vi "First Step.vi"(8 "error in (no error)":errorcluster, 11 "Magnetic Field Lakeshore Continuous.lvclass in":refnum<class "Magnetic Field Lakeshore Continuous.lvclass">) -> (0 "error out":errorcluster, 2 "Current Position":dbl, 3 "Magnetic Field Lakeshore Continuous.lvclass out":refnum<class "Magnetic Field Lakeshore Continuous.lvclass">)   [LabVIEW 2023, in "Magnetic Field Lakeshore Continuous.lvclass"]
doc: "(Dynamic) Reset the instrument and prepare to scan. Go to step #0 - the first step. If desired, the scanner may do this in a different way than usual (i.e. by preparing to move a long distance, or reset to home position.)"
uses:
  Magnetic Field Lakeshore Continuous.lvclass
  Magnetic Field Lakeshore Continuous.lvclass/Magnetic Field Lakeshore Continuous.ctl
  Scanner/Scanner.lvclass
  Instruments/Utility Classes/Scannable/Scannable.lvclass
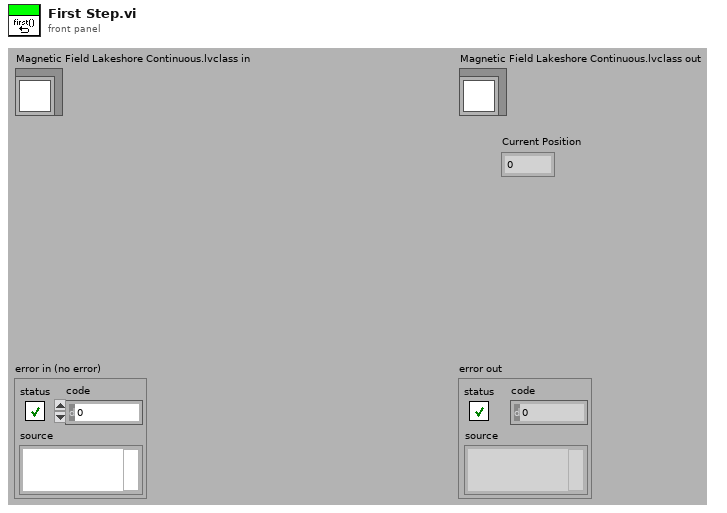
[diagram p1: front panel]
types:
  T1 = typedef "Scanner.lvclass/Range.ctl" = cluster{"xi":dbl, "xf":dbl, "dx":dbl, "Return to...?":bool, "Return to":dbl}
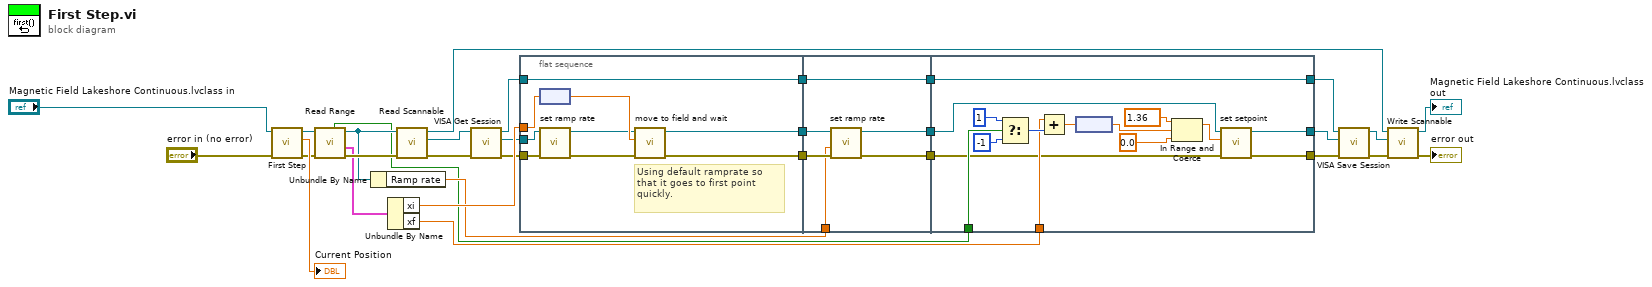
[diagram p0: block diagram]
diagram:
  n1 = call-parent "First Step.vi"("error in (no error)"="error in (no error)", "Scanner.lvclass in"="Magnetic Field Lakeshore Continuous.lvclass in") -> ("error out"=w27:errorcluster, "Current Position"=→"Current Position":dbl, "Scanner.lvclass out"=w28:refnum<class "Magnetic Field Lakeshore Continuous.lvclass">)  [unwired: 7 in]
  n2 = call-dynamic "Read Range.vi"("error in (no error)"=w27, "Scanner.lvclass in"=w28) -> ("error out"=w26:errorcluster, "Range"=w24:T1, "Scanner.lvclass out"=w25:refnum<class "Magnetic Field Lakeshore Continuous.lvclass">, "Scanning Up?"=w3:bool)  [unwired: 6 out]
  n3 = Unbundle By Name(w25) -> ("Ramp rate"=w4:dbl[unit])
  n4 = Unbundle By Name(w24) -> ("xi"=w16:dbl, "xf"=w2:dbl)
  n5 = call-dynamic "Read Scannable.vi"("error in (no error)"=w26, "Scanner.lvclass in"=w25) -> ("error out"=w10:errorcluster, "Scannable.lvclass"=w11:refnum<class "Scannable.lvclass">, "Scanner.lvclass out"=w21:refnum<class "Magnetic Field Lakeshore Continuous.lvclass">)  [unwired: 7 in]
  n6 = call-dynamic "VISA Get Session.vi"("error in (no error)"=w10, "Instrument.lvclass in"=w11) -> ("error out"=w8:errorcluster, "VISA Resource Name"=w7:refnum<visa-resource-name>, "Instrument.lvclass out"=w9:refnum<class "Scannable.lvclass">)  [unwired: 7 out]
  n7 = flat-sequence {
    tunnel: [w39] -> w22
    tunnel: w9 -> [w39]
    tunnel: [w37] -> w17
    tunnel: w8 -> [w33]
    tunnel: w16 -> [w40]
    tunnel: w7 -> [w35]
    tunnel: [w36] -> w6
    tunnel: [w46] -> w23
    tunnel: w22 -> [w46]
    tunnel: [w43] -> w18
    tunnel: w17 -> [w44]
    tunnel: w6 -> [w45]
    tunnel: [w42] -> w5
    tunnel: w4 -> [w41]
    tunnel: [w61] -> w15
    tunnel: w23 -> [w61]
    tunnel: [w47] -> w12
    tunnel: w18 -> [w48]
    tunnel: w5 -> [w50]
    tunnel: w3 -> [w58]
    tunnel: w2 -> [w56]
    tunnel: [w49] -> w1
    frame #0 {
      # "Using default ramprate so that it goes to first point quickly."
      n8 = node(w40) -> (w38:dbl[unit])
      n9 = call "set ramp rate.vi"("error in (no error)"=w33, "VISA session"=w35) -> ("error out"=w32:errorcluster, "dup VISA session"=w34:refnum<visa-resource-name>)  [unwired: 8 in]
      n10 = call "move to field and wait.vi"("error in (no error)"=w32, "Setpoint"=w38, "VISA session"=w34) -> ("error out"=w37:errorcluster, "dup VISA session"=w36:refnum<visa-resource-name>)  [unwired: 7 in]
    }
    frame #1 {
      n11 = call "set ramp rate.vi"("error in (no error)"=w44, "Ramp rate (3500 Gs/min)"=w41, "VISA session"=w45) -> ("error out"=w43:errorcluster, "dup VISA session"=w42:refnum<visa-resource-name>)  [unwired: 7 in]
    }
    frame #2 {
      n12 = Select(t=1, s=w58, f=-1) -> (s? t:f=w57:i32)
      n13 = Add(x=w56, y=w57) -> (x+y=w55:dbl)
      n14 = node(w55) -> (w54:dbl[unit])
      n15 = In Range and Coerce(upper limit=dbl[unit] 1.36, x=w54, lower limit=dbl[unit] 0.0) -> (coerced(x)=w51:dbl[unit])  [unwired: 1 out]
      n16 = call "set setpoint.vi"("error in (no error)"=w48, "Setpoint"=w51, "VISA session"=w50) -> ("error out"=w47:errorcluster, "dup VISA session"=w49:refnum<visa-resource-name>)  [unwired: 7 in]
    }
  }
  n17 = call-dynamic "VISA Save Session.vi"("error in (no error)"=w12, "VISA Resource Name"=w1, "Instrument.lvclass in"=w15) -> ("error out"=w13:errorcluster, "Instrument.lvclass out"=w14:refnum<class "Scannable.lvclass">)  [unwired: 7 out]
  n18 = call-dynamic "Write Scannable.vi"("error in (no error)"=w13, "Scannable.lvclass"=w14, "Scanner.lvclass in"=w21) -> ("error out"=→"error out":errorcluster, "Scanner.lvclass out"=→"Magnetic Field Lakeshore Continuous.lvclass out":refnum<class "Magnetic Field Lakeshore Continuous.lvclass">)  [unwired: 7 in]
